vi "output_buffer.vi"(0 "Line active":bool, 1 "Line out":bool, 2 "Out pin":refnum<k21>) -> ()   [LabVIEW 2011]
uses:
  <vilib>/rvi/eio/common/nirviEmuTemplateMethod_errors.vi
  <vilib>/eio/EIONode/EIONode.xnode
  <vilib>/eio/EIOMethodNode/EIOMethodNode.xnode
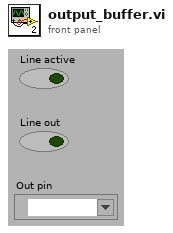
[diagram p1: front panel]
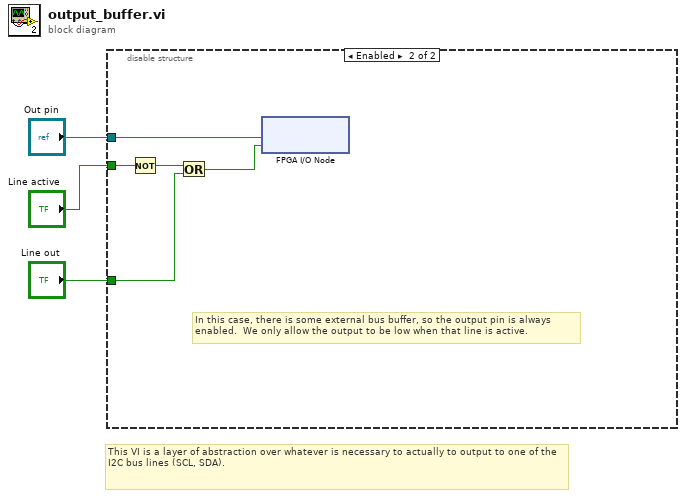
[diagram p0: block diagram]
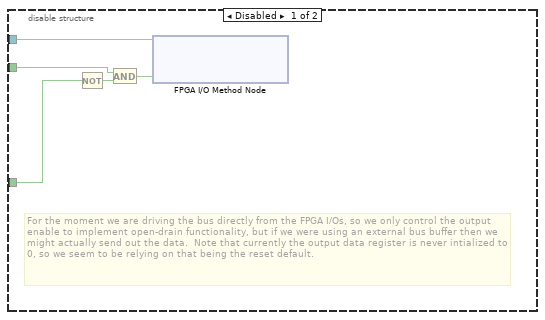
[diagram p2: hidden frame]
diagram:
  # "This VI is a layer of abstraction over whatever is necessary to actually to output to one of the I2C bus lines (SCL, SDA)."
  n1 = disable-structure shown="Enabled" {
    disable-tunnel: "Line active" -> [w7 w10]
    disable-tunnel: "Line out" -> [w6 w11]
    disable-tunnel: "Out pin" -> [w4 w13]
    frame Disabled {
      # "For the moment we are driving the bus directly from the FPGA I/Os, so we only control the output enable to implement open-drain functionality, but if we were using an external bus buffer then we might actually send out the data.  Note that currently the output data register is never intialized to 0, so we seem to be relying on that being the reset default."
      n2 = Not(x=w6) -> (.not. x?=w5:bool)
      n3 = And(x=w7, y=w5) -> (x .and. y?=w8:bool)
      n4 = xnode "FPGA I/O Method Node"("FPGA I/O In"=w4, "Enable"=w8) -> ()  [unwired: 1 out]
    }
    frame Enabled {
      # "In this case, there is some external bus buffer, so the output pin is always \nenabled.  We only allow the output to be low when that line is active."
      n5 = Not(x=w10) -> (.not. x?=w9:bool)
      n6 = Or(x=w9, y=w11) -> (x .or. y?=w12:bool)
      n7 = xnode "FPGA I/O Node"("I/O Item"=w12, "FPGA I/O In"=w13) -> ()  [unwired: 1 out]
    }
  }
